vi "GetTerms4.vi"(0 "XRef":T11, 1 "State In":T10) -> (14 "Terms":T2, 15 "Fatal Error Out":T1)   [LabVIEW 2015, in "LVJSON.lvlib" / "Index JSON Array.xnode"]
uses:
  Index JSON Array.xnode
  <vilib>/XNodeSupport/XNodeXNodeRef.ctl
  State.ctl
  <vilib>/XNodeSupport/XNodeTerm4Array.ctl
  <vilib>/XNodeSupport/XNodeTerm4.ctl
  <vilib>/XNodeSupport/XNodeString.ctl
  <vilib>/XNodeSupport/XNodeVariant.ctl
  <vilib>/XNodeSupport/XNodeRect32.ctl
  <vilib>/XNodeSupport/XNodeInt.ctl
  <vilib>/XNodeSupport/XNodeBool.ctl
  <vilib>/XNodeSupport/XNodeTermDirection.ctl
  <vilib>/XNodeSupport/XNodeErrorCluster.ctl
  JSON Datatype/JSON Null.lvclass
  dimensions.vi
  <vilib>/XNodeSupport/NI_XNodeSupport.lvlib
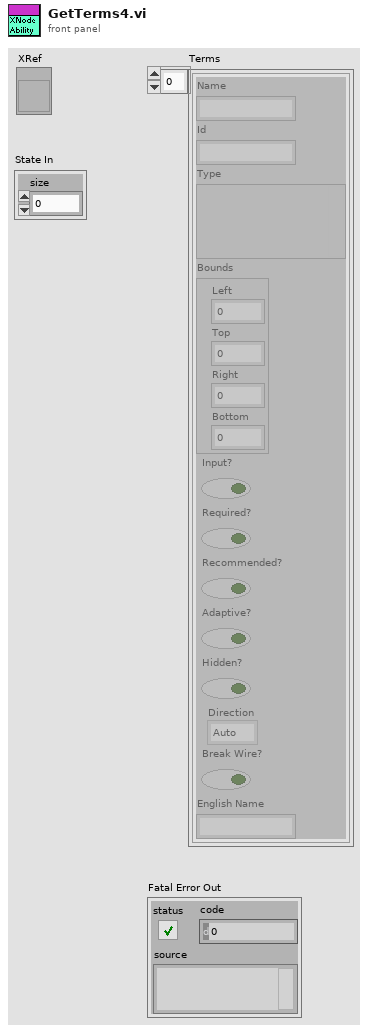
[diagram p1: front panel]
types:
  T1 = typedef "NI_XNodeSupport.lvlib/XNodeErrorCluster.ctl" = errorcluster
  T2 = typedef "NI_XNodeSupport.lvlib/XNodeTerm4Array.ctl" = T3[]
  T3 = typedef "NI_XNodeSupport.lvlib/XNodeTerm4.ctl" = cluster{"Name":T4, "Id":T4, "Type":T5, "Bounds":T6, "Input?":T8, "Required?":T8, "Recommended?":T8, "Adaptive?":T8, "Hidden?":T8, "Direction":T9, "Break Wire?":T8, "English Name":T4}
  T4 = typedef "NI_XNodeSupport.lvlib/XNodeString.ctl" = string
  T5 = typedef "NI_XNodeSupport.lvlib/XNodeVariant.ctl" = variant
  T6 = typedef "NI_XNodeSupport.lvlib/XNodeRect32.ctl" = cluster{"Left":T7, "Top":T7, "Right":T7, "Bottom":T7}
  T7 = typedef "NI_XNodeSupport.lvlib/XNodeInt.ctl" = i32
  T8 = typedef "NI_XNodeSupport.lvlib/XNodeBool.ctl" = bool
  T9 = typedef "NI_XNodeSupport.lvlib/XNodeTermDirection.ctl" = enum32{"Auto", "Up", "Down", "Left", "Right", "Center"}
  T10 = typedef "LVJSON.lvlib/Index JSON Array.xnode/State.ctl" = cluster{"size":u32}
  T11 = typedef "NI_XNodeSupport.lvlib/XNodeXNodeRef.ctl" = refnum<vi>
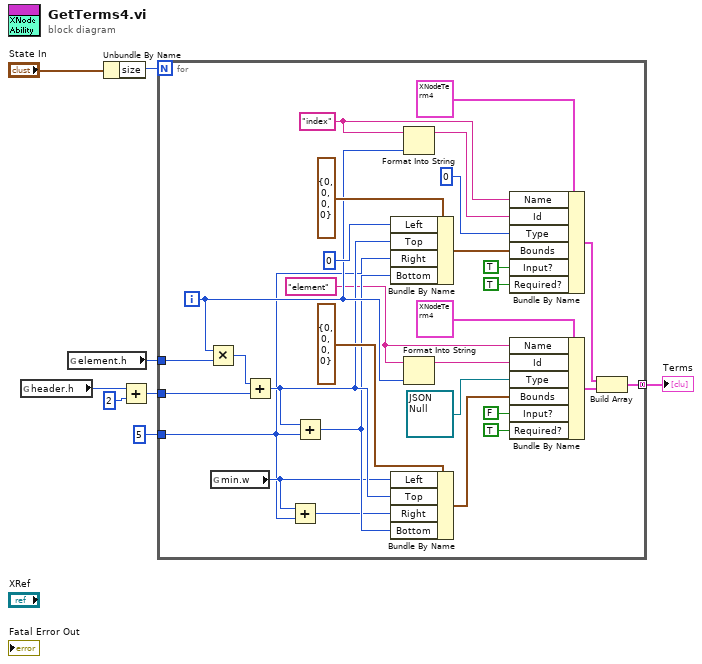
[diagram p0: block diagram]
diagram:
  n1 = global read "dimensions.vi" "header.h"() -> (w4:i16)
  n2 = global read "dimensions.vi" "element.h"() -> (w7:i16)
  n3 = Unbundle By Name("State In") -> ("size"=w6:u32)
  n4 = Add(x=w4, y=2) -> (x+y=w2:i32)
  n5 = for {
    N: w6 -> [_]
    tunnel: w7 -> [w31]
    tunnel: w2 -> [w28]
    tunnel: T7 5 ("Right") -> [w14]
    tunnel: [w11] -> w1 mode=concatenating
    i -> [w19]
    w9 = "element" ("initial string")
    w10 = "index" ("initial string")
    n6 = Multiply(x=w19, y=w31) -> (x*y=w29:i32)
    n7 = global read "dimensions.vi" "min.w"() -> (w15:i32)
    n8 = Add(x=w29, y=w28) -> (x+y=w17:i32)
    n9 = Add(x=w15, y=w14) -> (x+y=w13:T7)
    n10 = Add(x=w17, y=w14) -> (x+y=w16:T7)
    n11 = Bundle By Name(cluster=T6 {"Left"=0, "Top"=0, "Right"=0, "Bottom"=0} ("Bounds"), "Left"=T7 0, "Top"=w17, "Right"=w14, "Bottom"=w16) -> (w30:T6)
    n12 = Bundle By Name(cluster=T6 {"Left"=0, "Top"=0, "Right"=0, "Bottom"=0} ("Bounds"), "Left"=w15, "Top"=w17, "Right"=w13, "Bottom"=w16) -> (w25:T6)
    n13 = Format Into String(initial string=w10, w19) -> (resulting string=w36:string)  [unwired: 2 in, 1 out]
    n14 = Format Into String(initial string=w9, w19) -> (resulting string=w21:string)  [unwired: 2 in, 1 out]
    n15 = Bundle By Name(cluster=T3 {"Name"="", "Id"="", "Type"=variant, "Bounds"={"Left"=0, "Top"=0, "Right"=0, "Bottom"=0}, "Input?"=FALSE, "Required?"=FALSE, "Recommended?"=FALSE, "Adaptive?"=FALSE, "Hidden?"=FALSE, "Direction"=enum."Auto", "Break Wire?"=FALSE, "English Name"=""} ("Term 4"), "Name"=w10, "Id"=w36, "Type"=0 ("index"), "Bounds"=w30, "Input?"=T8 TRUE, "Required?"=T8 TRUE) -> (w26:T3)
    n16 = Bundle By Name(cluster=T3 {"Name"="", "Id"="", "Type"=variant, "Bounds"={"Left"=0, "Top"=0, "Right"=0, "Bottom"=0}, "Input?"=FALSE, "Required?"=FALSE, "Recommended?"=FALSE, "Adaptive?"=FALSE, "Hidden?"=FALSE, "Direction"=enum."Auto", "Break Wire?"=FALSE, "English Name"=""} ("Term 4"), "Name"=w9, "Id"=w21, "Type"=refnum<class "JSON Null.lvclass"> refnum ("LVJSON.lvlib:JSON Null.lvclass"), "Bounds"=w25, "Input?"=T8 FALSE, "Required?"=T8 TRUE) -> (w12:T3)
    n17 = Build Array(w26, w12) -> (w11:T3[])
  }
  "Terms" <- w1
